vi "IT6932A_set voltage current.vi"(4 "Current":i32, 6 "Voltage":i32, 8 "error in (no error)":errorcluster, 10 "On/Off":bool, 11 "VISA resource name 4":refnum<visa-resource-name>) -> (1 "error out":errorcluster)   [LabVIEW 2023]
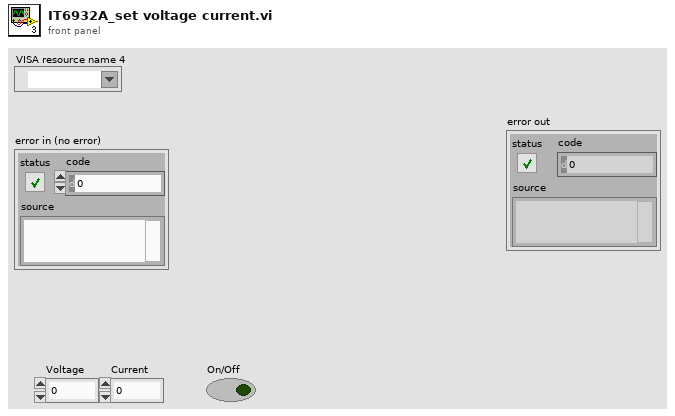
[diagram p1: front panel]
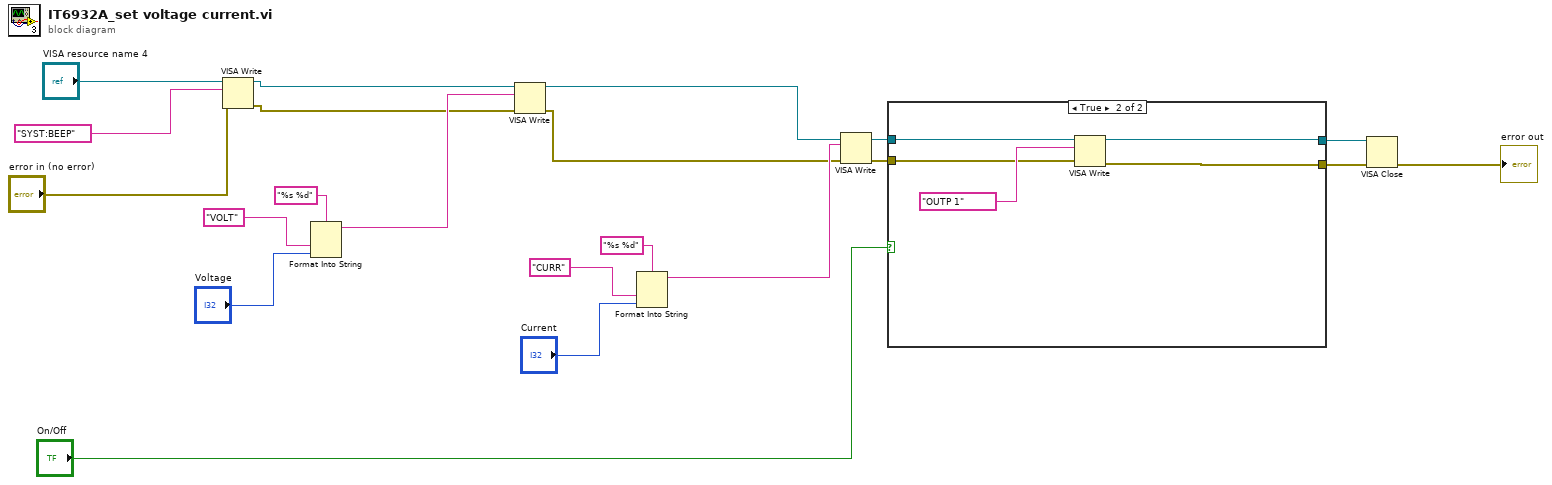
[diagram p0: block diagram]
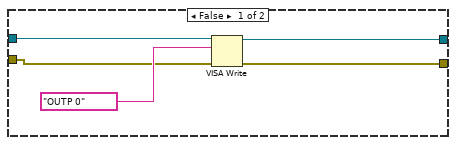
[diagram p2: hidden frame]
diagram:
  n1 = VISA Write(VISA resource name="VISA resource name 4", write buffer="SYST:BEEP", error in (no error)="error in (no error)") -> (VISA resource name out=w12:refnum<visa-resource-name>, error out=w8:errorcluster)  [unwired: 1 out]
  n2 = Format Into String(format string="%s %d", "VOLT" ("write buffer"), "Voltage") -> (resulting string=w17:string)  [unwired: 2 in, 1 out]
  n3 = VISA Write(VISA resource name=w12, write buffer=w17, error in (no error)=w8) -> (VISA resource name out=w11:refnum<visa-resource-name>, error out=w7:errorcluster)  [unwired: 1 out]
  n4 = Format Into String(format string="%s %d", "CURR" ("write buffer"), "Current") -> (resulting string=w10:string)  [unwired: 2 in, 1 out]
  n5 = VISA Write(VISA resource name=w11, write buffer=w10, error in (no error)=w7) -> (VISA resource name out=w9:refnum<visa-resource-name>, error out=w6:errorcluster)  [unwired: 1 out]
  n6 = case shown="True" "On/Off" {
    tunnel: w9 -> [w25 w31]
    tunnel: w6 -> [w24 w29]
    tunnel: [w23 w28] -> w2
    tunnel: [w22 w27] -> w3
    frame False {
      n7 = VISA Write(VISA resource name=w25, write buffer="OUTP 0", error in (no error)=w24) -> (VISA resource name out=w22:refnum<visa-resource-name>, error out=w23:errorcluster)  [unwired: 1 out]
    }
    frame True {
      n8 = VISA Write(VISA resource name=w31, write buffer="OUTP 1", error in (no error)=w29) -> (VISA resource name out=w27:refnum<visa-resource-name>, error out=w28:errorcluster)  [unwired: 1 out]
    }
  }
  n9 = VISA Close(VISA resource name=w3, error in (no error)=w2) -> (error out=→"error out":errorcluster)
